vi "Func-엑셀 데이터를 그래프로 출력.vi"() -> ()   [LabVIEW 2015] (continued)
\n-40\t-40\t-28.416\n-40\t-40\t-28.418\n-40\t-40\t-28.417\n-40\t-40\t-28.42\n-40\t-40\t-28.421\n-40\t-40\t-28.421\n-40\t-40\t-28.429\n-40\t-40\t-28.43\n-40\t-40\t-28.434\n-40\t-40\t-28.438\n-40\t-40\t-28.439\n-40\t-40\t-28.439\n-40\t-40\t-28.438\n-40\t-40\t-28.443\n-40\t-40\t-28.445\n-40\t-40\t-28.446\n-40\t-40\t-28.45\n-40\t-40\t-28.455\n-40\t-40\t-28.458\n-40\t-40\t-28.458\n-40\t-40\t-28.46\n-40\t-40\t-28.465\n-40\t-40\t-28.466\n-40\t-40\t-28.466\n-40\t-40\t-28.471\n-40\t-40\t-28.47\n-40\t-40\t-28.475\n-40\t-40\t-28.474\n-40\t-40\t-28.476\n-40\t-40\t-28.478\n-40\t-40\t-28.48\n-40\t-40\t-28.48\n-40\t-40\t-28.479\n-40\t-40\t-28.485\n-40\t-40\t-28.484\n-40\t-40\t-28.488\n-40\t-40\t-28.494\n-40\t-40\t-28.498\n-40\t-40\t-28.499\n-40\t-40\t-28.499\n-40\t-40\t-28.502\n-40\t-40\t-28.504\n-40\t-40\t-28.504\n-40\t-40\t-28.507\n-40\t-40\t-28.508\n-40\t-40\t-28.514\n-40\t-40\t-28.518\n-40\t-40\t-28.52\n-40\t-40\t-28.523\n-40\t-40\t-28.524\n-40\t-40\t-28.53\n-40\t-40\t-28.534\n-40\t-40\t-28.536\n-40\t-40\t-28.539\n-40\t-40\t-28.543\n-40\t-40\t-28.544\n-40\t-40\t-28.544\n-40\t-40\t-28.542\n-40\t-40\t-28.542\n-40\t-40\t-28.542\n-40\t-40\t-28.544\n-40\t-40\t-28.548\n-40\t-40\t-28.55\n-40\t-40\t-28.553\n-40\t-40\t-28.552\n-40\t-40\t-28.554\n-40\t-40\t-28.555\n-40\t-40\t-28.557\n-40\t-40\t-28.557\n-40\t-40\t-28.559\n-40\t-40\t-28.564\n-40\t-40\t-28.57\n-40\t-40\t-28.57\n-40\t-40\t-28.57\n-40\t-40\t-28.574\n-40\t-40\t-28.578\n-40\t-40\t-28.58\n-40\t-40\t-28.577\n-40\t-40\t-28.581\n-40\t-40\t-28.585\n-40\t-40\t-28.586\n-40\t-40\t-28.588\n-40\t-40\t-28.587\n-40\t-40\t-28.593\n-40\t-40\t-28.593\n-40\t-40\t-28.593\n-40\t-40\t-28.594\n-40\t-40\t-28.596\n-40\t-40\t-28.602\n-40\t-40\t-28.605\n-40\t-40\t-28.611\n-40\t-40\t-28.614\n-40\t-40\t-28.617\n-40\t-40\t-28.621\n-40\t-40\t-28.62\n-40\t-40\t-28.62\n-40\t-40\t-28.618\n-40\t-40\t-28.618\n-40\t-40\t-28.62\n-40\t-40\t-28.62\n-40\t-40\t-28.625\n-40\t-40\t-28.629\n-40\t-40\t-28.634\n-40\t-40\t-28.635\n-40\t-40\t-28.636\n-40\t-40\t-28.639\n-40\t-40\t-28.639\n-40\t-40\t-28.643\n-40\t-40\t-28.643\n-40\t-40\t-28.646\n-40\t-40\t-28.65\n-40\t-40\t-28.652\n-40\t-40\t-28.653\n-40\t-40\t-28.654\n-40\t-40\t-28.656\n-40\t-40\t-28.655\n-40\t-40\t-28.655\n-40\t-40\t-28.657\n-40\t-40\t-28.658\n-40\t-40\t-28.662\n-40\t-40\t-28.662\n-40\t-40\t-28.666\n-40\t-40\t-28.67\n-40\t-40\t-28.674\n-40\t-40\t-28.676\n-40\t-40\t-28.677\n-40\t-40\t-28.679\n-40\t-40\t-28.684\n-40\t-40\t-28.687\n-40\t-40\t-28.687\n-40\t-40\t-28.688\n-40\t-40\t-28.692\n-40\t-40\t-28.691\n-40\t-40\t-28.69\n-40\t-40\t-28.692\n-40\t-40\t-28.695\n-40\t-40\t-28.697\n-40\t-40\t-28.695\n-40\t-40\t-28.7\n-40\t-40\t-28.703\n-40\t-40\t-28.708\n-40\t-40\t-28.708\n-40\t-40\t-28.709\n-40\t-40\t-28.716\n-40\t-40\t-28.72\n-40\t-40\t-28.72\n-40\t-40\t-28.718\n-40\t-40\t-28.721\n-40\t-40\t-28.724\n-40\t-40\t-28.726\n-40\t-40\t-28.728\n-40\t-40\t-28.731\n-40\t-40\t-28.733\n-40\t-40\t-28.732\n-40\t-40\t-28.731\n-40\t-40\t-28.731\n-40\t-40\t-28.73\n-40\t-40\t-28.732\n-40\t-40\t-28.736\n-40\t-40\t-28.739\n-40\t-40\t-28.742\n-40\t-40\t-28.745\n-40\t-40\t-28.746\n-40\t-40\t-28.748\n-40\t-40\t-28.75\n-40\t-40\t-28.751\n-40\t-40\t-28.752\n-40\t-40\t-28.754\n-40\t-40\t-28.755\n-40\t-40\t-28.757\n-40\t-40\t-28.758\n-40\t-40\t-28.761\n-40\t-40\t-28.762\n-40\t-40\t-28.764\n-40\t-40\t-28.767\n-40\t-40\t-28.769\n-40\t-40\t-28.772\n-40\t-40\t-28.774\n-40\t-40\t-28.778\n-40\t-40\t-28.775\n-40\t-40\t-28.778\n-40\t-40\t-28.78\n-40\t-40\t-28.781\n-40\t-40\t-28.781\n-40\t-40\t-28.784\n-40\t-40\t-28.791\n-40\t-40\t-28.793\n-40\t-40\t-28.793\n-40\t-40\t-28.799\n-40\t-40\t-28.8\n-40\t-40\t-28.801\n-40\t-40\t-28.802\n-40\t-40\t-28.804\n-40\t-40\t-28.803\n-40\t-40\t-28.805\n-40\t-40\t-28.806\n-40\t-40\t-28.807\n-40\t-40\t-28.808\n-40\t-40\t-28.809\n-40\t-40\t-28.813\n-40\t-40\t-28.812\n-40\t-40\t-28.815\n-40\t-40\t-28.819\n-40\t-40\t-28.823\n-40\t-40\t-28.821\n-40\t-40\t-28.824\n-40\t-40\t-28.826\n-40\t-40\t-28.827\n-40\t-40\t-28.829\n-40\t-40\t-28.831\n-40\t-40\t-28.837\n-40\t-40\t-28.839\n-40\t-40\t-28.844\n-40\t-40\t-28.845\n-40\t-40\t-28.848\n-40\t-40\t-28.85\n-40\t-40\t-28.848\n-40\t-40\t-28.848\n-40\t-40\t-28.846\n-40\t-40\t-28.85\n-40\t-40\t-28.851\n-40\t-40\t-28.848\n-40\t-40\t-28.851\n-40\t-40\t-28.851\n-40\t-40\t-28.855\n-40\t-40\t-28.855\n-40\t-40\t-28.856\n-40\t-40\t-28.861\n-40\t-40\t-28.862\n-40\t-40\t-28.867\n-40\t-40\t-28.868\n-40\t-40\t-28.871\n-40\t-40\t-28.871\n-40\t-40\t-28.873\n-40\t-40\t-28.873\n-40\t-40\t-28.874\n-40\t-40\t-28.876\n-40\t-40\t-28.875\n-40\t-40\t-28.879\n-40\t-40\t-28.881\n-40\t-40\t-28.881\n-40\t-40\t-28.886\n-40\t-40\t-28.888\n-40\t-40\t-28.892\n-40\t-40\t-28.891\n-40\t-40\t-28.893\n-40\t-40\t-28.899\n-40\t-40\t-28.895\n-40\t-40\t-28.897\n-40\t-40\t-28.899\n-40\t-40\t-28.905\n-40\t-40\t-28.906\n-40\t-40\t-28.905\n-40\t-40\t-28.911\n-40\t-40\t-28.911\n-40\t-40\t-28.911\n-40\t-40\t-28.911\n-40\t-40\t-28.913\n-40\t-40\t-28.918\n-40\t-40\t-28.918\n-40\t-40\t-28.919\n-40\t-40\t-28.919\n-40\t-40\t-28.923\n-40\t-40\t-28.924\n-40\t-40\t-28.924\n-40\t-40\t-28.926\n-40\t-40\t-28.929\n-40\t-40\t-28.932\n-40\t-40\t-28.931\n-40\t-40\t-28.931\n-40\t-40\t-28.932\n-40\t-40\t-28.935\n-40\t-40\t-28.936\n-40\t-40\t-28.938\n-40\t-40\t-28.941\n-40\t-40\t-28.943\n-40\t-40\t-28.945\n-40\t-40\t-28.943\n-40\t-40\t-28.945\n-40\t-40\t-28.943\n-40\t-40\t-28.942\n-40\t-40\t-28.943\n-40\t-40\t-28.943\n-40\t-40\t-28.948\n-40\t-40\t-28.946\n-40\t-40\t-28.948\n-40\t-40\t-28.955\n-40\t-40\t-28.955\n-40\t-40\t-28.958\n-40\t-40\t-28.959\n-40\t-40\t-28.965\n-40\t-40\t-28.969\n-40\t-40\t-28.966\n-40\t-40\t-28.971\n-40\t-40\t-28.971\n-40\t-40\t-28.974\n-40\t-40\t-28.974\n-40\t-40\t-28.974\n-40\t-40\t-28.971\n-40\t-40\t-28.968\n-40\t-40\t-28.971\n-40\t-40\t-28.974\n-40\t-40\t-28.975\n-40\t-40\t-28.977\n-40\t-40\t-28.987\n-40\t-40\t-28.994\n-40\t-40\t-28.995\n-40\t-40\t-28.996\n-40\t-40\t-28.997\n-40\t-40\t-29\n-40\t-40\t-29.003\n-40\t-40\t-29.003\n-40\t-40\t-29.003\n-40\t-40\t-29.002\n-40\t-40\t-29.004\n-40\t-40\t-29.003\n-40\t-40\t-29.003\n-40\t-40\t-29.005\n-40\t-40\t-29.006\n-40\t-40\t-29.01\n-40\t-40\t-29.009\n-40\t-40\t-29.01\n-40\t-40\t-29.009\n-40\t-40\t-29.007\n-40\t-40\t-29.007\n-40\t-40\t-29.011\n-40\t-40\t-29.015\n-40\t-40\t-29.018\n-40\t-40\t-29.02\n-40\t-40\t-29.022\n-40\t-40\t-29.024\n-40\t-40\t-29.024\n-40\t-40\t-29.024\n-40\t-40\t-29.025\n-40\t-40\t-29.03\n-40\t-40\t-29.035\n-40\t-40\t-29.036\n-40\t-40\t-29.033\n-40\t-40\t-29.031\n-40\t-40\t-29.031\n-40\t-40\t-29.034\n-40\t-40\t-29.032\n-40\t-40\t-29.033\n-40\t-40\t-29.037\n-40\t-40\t-29.04\n-40\t-40\t-29.043\n-40\t-40\t-29.047\n-40\t-40\t-29.047\n-40\t-40\t-29.048\n-40\t-40\t-29.053\n-40\t-40\t-29.055\n-40\t-40\t-29.055\n-40\t-40\t-29.055\n-40\t-40\t-29.059\n-40\t-40\t-29.062\n-40\t-40\t-29.063\n-40\t-40\t-29.066\n-40\t-40\t-29.067\n-40\t-40\t-29.067\n-40\t-40\t-29.066\n-40\t-40\t-29.066\n-40\t-40\t-29.071\n-40\t-40\t-29.075\n-40\t-40\t-29.075\n-40\t-40\t-29.076\n-40\t-40\t-29.079\n-40\t-40\t-29.082\n-40\t-40\t-29.079\n-40\t-40\t-29.078\n-40\t-40\t-29.079\n-40\t-40\t-29.079\n-40\t-40\t-29.08\n-40\t-40\t-29.08\n-40\t-40\t-29.08\n-40\t-40\t-29.081\n-40\t-40\t-29.084\n-40\t-40\t-29.09\n-40\t-40\t-29.091\n-40\t-40\t-29.091\n-40\t-40\t-29.098\n-40\t-40\t-29.096\n-40\t-40\t-29.099\n-40\t-40\t-29.096\n-40\t-40\t-29.098\n-40\t-40\t-29.1\n-40\t-40\t-29.101\n-40\t-40\t-29.106\n-40\t-40\t-29.108\n-40\t-40\t-29.111\n-40\t-40\t-29.114\n-40\t-40\t-29.117\n-40\t-40\t-29.12\n-40\t-40\t-29.119\n-40\t-40\t-29.121\n-40\t-40\t-29.123\n-40\t-40\t-29.121\n-40\t-40\t-29.12\n-40\t-40\t-29.121\n-40\t-40\t-29.123\n-40\t-40\t-29.12\n-40\t-40\t-29.123\n-40\t-40\t-29.126\n-40\t-40\t-29.128\n-40\t-40\t-29.129\n-40\t-40\t-29.129\n-40\t-40\t-29.132\n-40\t-40\t-29.133\n-40\t-40\t-29.134\n-40\t-40\t-29.136\n-40\t-40\t-29.138\n-40\t-40\t-29.137\n-40\t-40\t-29.139\n-40\t-40\t-29.142\n-40\t-40\t-29.141\n-40\t-40\t-29.142\n-40\t-40\t-29.143\n-40\t-40\t-29.146\n-40\t-40\t-29.145\n-40\t-40\t-29.146\n-40\t-40\t-29.148\n-40\t-40\t-29.148\n-40\t-40\t-29.151\n-40\t-40\t-29.15\n-40\t-40\t-29.152\n-40\t-40\t-29.149\n-40\t-40\t-29.153\n-40\t-40\t-29.157\n-40\t-40\t-29.155\n-40\t-40\t-29.161\n-40\t-40\t-29.163\n-40\t-40\t-29.165\n-40\t-40\t-29.165\n-40\t-40\t-29.164\n-40\t-40\t-29.166\n-40\t-40\t-29.162\n-40\t-40\t-29.161\n-40\t-40\t-29.166\n-40\t-40\t-29.168\n-40\t-40\t-29.169\n-40\t-40\t-29.171\n-40\t-40\t-29.175\n-40\t-40\t-29.177\n-40\t-40\t-29.177\n-40\t-40\t-29.18\n-40\t-40\t-29.182\n-40\t-40\t-29.184\n-40\t-40\t-29.186\n-40\t-40\t-29.187\n-40\t-40\t-29.186\n-40\t-40\t-29.186\n-40\t-40\t-29.19\n-40\t-40\t-29.193\n-40\t-40\t-29.191\n-40\t-40\t-29.191\n-40\t-40\t-29.197\n-40\t-40\t-29.197\n-40\t-40\t-29.196\n-40\t-40\t-29.196\n-40\t-40\t-29.2\n-40\t-40\t-29.2\n-40\t-40\t-29.2\n-40\t-40\t-29.199\n-40\t-40\t-29.199\n-40\t-40\t-29.202\n-40\t-40\t-29.202\n-40\t-40\t-29.206\n-40\t-40\t-29.205\n-40\t-40\t-29.208\n-40\t-40\t-29.208\n-40\t-40\t-29.209\n-40\t-40\t-29.211\n-40\t-40\t-29.211\n-40\t-40\t-29.213\n-40\t-40\t-29.215\n-40\t-40\t-29.22\n-40\t-40\t-29.221\n-40\t-40\t-29.226\n-40\t-40\t-29.226\n-40\t-40\t-29.23\n-40\t-40\t-29.231\n-40\t-40\t-29.229\n-40\t-40\t-29.229\n-40\t-40\t-29.226\n-40\t-40\t-29.229\n-40\t-40\t-29.23\n-40\t-40\t-29.232\n-40\t-40\t-29.233\n-40\t-40\t-29.238\n-40\t-40\t-29.24\n-40\t-40\t-29.24\n-40\t-40\t-29.241\n-40\t-40\t-29.241\n-40\t-40\t-29.241\n-40\t-40\t-29.243\n-40\t-40\t-29.243\n-40\t-40\t-29.247\n-40\t-40\t-29.251\n-40\t-40\t-29.251\n-40\t-40\t-29.254\n-40\t-40\t-29.252\n-40\t-40\t-29.252\n-40\t-40\t-29.253\n-40\t-40\t-29.252\n-40\t-40\t-29.254\n-40\t-40\t-29.254\n-40\t-40\t-29.259\n-40\t-40\t-29.262\n-40\t-40\t-29.26\n-40\t-40\t-29.259\n-40\t-40\t-29.259\n-40\t-40\t-29.261\n-40\t-40\t-29.26\n-40\t-40\t-29.261\n-40\t-40\t-29.262\n-40\t-40\t-29.267\n-40\t-40\t-29.27\n-40\t-40\t-29.27\n-40\t-40\t-29.27\n-40\t-40\t-29.273\n-40\t-40\t-29.273\n-40\t-40\t-29.273\n-40\t-40\t-29.275\n-40\t-40\t-29.277\n-40\t-40\t-29.279\n-40\t-40\t-29.277\n-40\t-40\t-29.284\n-40\t-40\t-29.286\n-40\t-40\t-29.285\n-40\t-40\t-29.288\n-40\t-40\t-29.291\n-40\t-40\t-29.289\n-40\t-40\t-29.288\n-40\t-40\t-29.284\n-40\t-40\t-29.284\n-40\t-40\t-29.283\n-40\t-40\t-29.282\n-40\t-40\t-29.284\n-40\t-40\t-29.286\n-40\t-40\t-29.29\n-40\t-40\t-29.294\n-40\t-40\t-29.298\n-40\t-40\t-29.302\n-40\t-40\t-29.303\n-40\t-40\t-29.302\n-40\t-40\t-29.301\n-40\t-40\t-29.3\n-40\t-40\t-29.297\n-40\t-40\t-29.295\n-40\t-40\t-29.297\n-40\t-40\t-29.3\n-40\t-40\t-29.307\n-40\t-40\t-29.307\n-40\t-40\t-29.309\n-40\t-40\t-29.312\n-40\t-40\t-29.313\n-40\t-40\t-29.312\n-40\t-40\t-29.309\n-40\t-40\t-29.313\n-40\t-40\t-29.314\n-40\t-40\t-29.318\n-40\t-40\t-29.32\n-40\t-40\t-29.32\n-40\t-40\t-29.325\n-40\t-40\t-29.325\n-40\t-40\t-29.327\n-40\t-40\t-29.327\n-40\t-40\t-29.329\n-40\t-40\t-29.33\n-40\t-40\t-29.327\n-40\t-40\t-29.326\n-40\t-40\t-29.325\n-40\t-40\t-29.326\n-40\t-40\t-29.328\n-40\t-40\t-29.329\n-40\t-40\t-29.332\n-40\t-40\t-29.332\n-40\t-40\t-29.337\n-40\t-40\t-29.339\n-40\t-40\t-29.339\n-40\t-40\t-29.34\n-40\t-40\t-29.343\n-40\t-40\t-29.347\n-40\t-40\t-29.345\n-40\t-40\t-29.346\n-40\t-40\t-29.348\n-40\t-40\t-29.351\n-40\t-40\t-29.349\n-40\t-40\t-29.346\n-40\t-40\t-29.347\n-40\t-40\t-29.349\n-40\t-40\t-29.349\n-40\t-40\t-29.35\n-40\t-40\t-29.356\n-40\t-40\t-29.359\n-40\t-40\t-29.357\n-40\t-40\t-29.356\n-40\t-40\t-29.355\n-40\t-40\t-29.358\n-40\t-40\t-29.359\n-40\t-40\t-29.362\n-40\t-40\t-29.365\n-40\t-40\t-29.37\n-40\t-40\t-29.368\n-40\t-40\t-29.365\n-40\t-40\t-29.364\n-40\t-40\t-29.365\n-40\t-40\t-29.369\n-40\t-40\t-29.363\n-40\t-40\t-29.366\n-40\t-40\t-29.367\n-40\t-40\t-29.37\n-40\t-40\t-29.37\n-40\t-40\t-29.37\n-40\t-40\t-29.376\n-40\t-40\t-29.378\n-40\t-40\t-29.38\n-40\t-40\t-29.383\n-40\t-40\t-29.385\n-40\t-40\t-29.381\n-40\t-40\t-29.382\n-40\t-40\t-29.385\n-40\t-40\t-29.385\n-40\t-40\t-29.384\n-40\t-40\t-29.383\n-40\t-40\t-29.386\n-40\t-40\t-29.386\n-40\t-40\t-29.386\n-40\t-40\t-29.387\n-40\t-40\t-29.389\n-40\t-40\t-29.39\n-40\t-40\t-29.392\n-40\t-40\t-29.393\n-40\t-40\t-29.393\n-40\t-40\t-29.396\n-40\t-40\t-29.4\n-40\t-40\t-29.404\n-40\t-40\t-29.401\n-40\t-40\t-29.401\n-40\t-40\t-29.404\n-40\t-40\t-29.401\n-40\t-40\t-29.398\n-40\t-40\t-29.397\n-40\t-40\t-29.399\n-40\t-40\t-29.402\n-40\t-40\t-29.4\n-40\t-40\t-29.405\n-40\t-40\t-29.41\n-40\t-40\t-29.413\n-40\t-40\t-29.413\n-40\t-40\t-29.413\n-40\t-40\t-29.413\n-40\t-40\t-29.411\n-40\t-40\t-29.41\n-40\t-40\t-29.409\n-40\t-40\t-29.41\n-40\t-40\t-29.414\n-40\t-40\t-29.415\n-40\t-40\t-29.416\n-40\t-40\t-29.418\n-40\t-40\t-29.419\n-40\t-40\t-29.421\n-40\t-40\t-29.42\n-40\t-40\t-29.423\n-40\t-40\t-29.424\n-40\t-40\t-29.422\n-40\t-40\t-29.423\n-40\t-40\t-29.424\n-40\t-40\t-29.423\n-40\t-40\t-29.423\n-40\t-40\t-29.424\n-40\t-40\t-29.43\n-40\t-40\t-29.431\n-40\t-40\t-29.43\n-40\t-40\t-29.434\n-40\t-40\t-29.435\n-40\t-40\t-29.438\n-40\t-40\t-29.436\n-40\t-40\t-29.44\n-40\t-40\t-29.441\n-40\t-40\t-29.441\n-40\t-40\t-29.444\n-40\t-40\t-29.442\n-40\t-40\t-29.442\n-40\t-40\t-29.441\n-40\t-40\t-29.443\n-40\t-40\t-29.446\n-40\t-40\t-29.446\n-40\t-40\t-29.447\n-40\t-40\t-29.454\n-40\t-40\t-29.452\n-40\t-40\t-29.452\n-40\t-40\t-29.454\n-40\t-40\t-29.454\n-40\t-40\t-29.456\n-40\t-40\t-29.452\n-40\t-40\t-29.452\n-40\t-40\t-29.455\n-40\t-40\t-29.455\n-40\t-40\t-29.453\n-40\t-40\t-29.453\n-40\t-40\t-29.457\n-40\t-40\t-29.46\n-40\t-40\t-29.459\n-40\t-40\t-29.462\n-40\t-40\t-29.464\n-40\t-40\t-29.464\n-40\t-40\t-29.466\n-40\t-40\t-29.467\n-40\t-40\t-29.468\n-40\t-40\t-29.47\n-40\t-40\t-29.471\n-40\t-40\t-29.474\n-40\t-40\t-29.474\n-40\t-40\t-29.473\n-40\t-40\t-29.476\n-40\t-40\t-29.472\n-40\t-40\t-29.473\n-40\t-40\t-29.472\n-40\t-40\t-29.471\n-40\t-40\t-29.473\n-40\t-40\t-29.473\n-40\t-40\t-29.475\n-40\t-40\t-29.477\n-40\t-40\t-29.477\n-40\t-40\t-29.475\n-40\t-40\t-29.476\n-40\t-40\t-29.475\n-40\t-40\t-29.474\n-40\t-40\t-29.474\n-40\t-40\t-29.476\n-40\t-40\t-29.481\n-40\t-40\t-29.484\n-40\t-40\t-29.485\n-40\t-40\t-29.49\n-40\t-40\t-29.493\n-40\t-40\t-29.492\n-40\t-40\t-29.496\n-40\t-40\t-29.498\n-40\t-40\t-29.498\n-40\t-40\t-29.5\n-40\t-40\t-29.5\n-40\t-40\t-29.501\n-40\t-40\t-29.496\n-40\t-40\t-29.493\n-40\t-40\t-29.495\n-40\t-40\t-29.495\n-40\t-40\t-29.494\n-40\t-40\t-29.496\n-40\t-40\t-29.498\n-40\t-40\t-29.499\n-40\t-40\t-29.498\n-40\t-40\t-29.499\n-40\t-40\t-29.5\n-40\t-40\t-29.502\n-40\t-40\t-29.501\n-40\t-40\t-29.502\n-40\t-40\t-29.501\n-40\t-40\t-29.5\n-40\t-40\t-29.5\n-40\t-40\t-29.501\n-40\t-40\t-29.502\n-40\t-40\t-29.507\n-40\t-40\t-29.51\n-40\t-40\t-29.509\n-40\t-40\t-29.511\n-40\t-40\t-29.512\n-40\t-40\t-29.513\n-40\t-40\t-29.51\n-40\t-40\t-29.511\n-40\t-40\t-29.512\n-40\t-40\t-29.514\n-40\t-40\t-29.514\n-40\t-40\t-29.516\n-40\t-40\t-29.516\n-40\t-40\t-29.516\n-40\t-40\t-29.523\n-40\t-40\t-29.521\n-40\t-40\t-29.521\n-40\t-40\t-29.523\n-40\t-40\t-29.524\n-40\t-40\t-29.526\n-40\t-40\t-29.522\n-40\t-40\t-29.522\n-40\t-40\t-29.526\n-40\t-40\t-29.529\n-40\t-40\t-29.531\n-40\t-40\t-29.534\n-40\t-40\t-29.536\n-40\t-40\t-29.54\n-40\t-40\t-29.539\n-40\t-40\t-29.539\n-40\t-40\t-29.543\n-40\t-40\t-29.536\n-40\t-40\t-29.539\n-40\t-40\t-29.542\n-40\t-40\t-29.542\n-40\t-40\t-29.542\n-40\t-40\t-29.541\n-40\t-40\t-29.543\n-40\t-40\t-29.539\n-40\t-40\t-29.538\n-40\t-40\t-29.541\n-40\t-40\t-29.54\n-40\t-40\t-29.54\n-40\t-40\t-29.544\n-40\t-40\t-29.549\n-40\t-40\t-29.55\n-40\t-40\t-29.548\n-40\t-40\t-29.552\n-40\t-40\t-29.551\n-40\t-40\t-29.553\n-40\t-40\t-29.55\n-40\t-40\t-29.552\n-40\t-40\t-29.554\n-40\t-40\t-29.554\n-40\t-40\t-29.555\n-40\t-40\t-29.554\n-40\t-40\t-29.558\n-40\t-40\t-29.561\n-40\t-40\t-29.56\n-40\t-40\t-29.562\n-40\t-40\t-29.561\n-40\t-40\t-29.56\n-40\t-40\t-29.556\n-40\t-40\t-29.556\n-40\t-40\t-29.556\n-40\t-40\t-29.556\n-40\t-40\t-29.558\n-40\t-40\t-29.559\n-40\t-40\t-29.561\n-40\t-40\t-29.557\n-40\t-40\t-29.56\n-40\t-40\t-29.558\n-40\t-40\t-29.561\n-40\t-40\t-29.563\n-40\t-40\t-29.566\n-40\t-40\t-29.57\n-40\t-40\t-29.57\n-40\t-40\t-29.573\n-40\t-40\t-29.575\n-40\t-40\t-29.576\n-40\t-40\t-29.573\n-40\t-40\t-29.573\n-40\t-40\t-29.571\n-40\t-40\t-29.567\n-40\t-40\t-29.568\n-40\t-40\t-29.568\n-40\t-40\t-29.572\n-40\t-40\t-29.578\n-40\t-40\t-29.58\n-40\t-40\t-29.587\n-40\t-40\t-29.585\n-40\t-40\t-29.587\n-40\t-40\t-29.586\n-40\t-40\t-29.584\n-40\t-40\t-29.585\n-40\t-40\t-29.584\n-40\t-40\t-29.586\n-40\t-40\t-29.585\n-40\t-40\t-29.584\n-40\t-40\t-29.582\n-40\t-40\t-29.581\n-40\t-40\t-29.582\n-40\t-40\t-29.585\n-40\t-40\t-29.586\n-40\t-40\t-29.591\n-40\t-40\t-29.598\n-40\t-40\t-29.597\n-40\t-40\t-29.598\n-40\t-40\t-29.599\n-40\t-40\t-29.601\n-40\t-40\t-29.6\n-40\t-40\t-29.598\n-40\t-40\t-29.601\n-40\t-40\t-29.602\n-40\t-40\t-29.602\n-40\t-40\t-29.601\n-40\t-40\t-29.601\n-40\t-40\t-29.602\n-40\t-40\t-29.603\n-40\t-40\t-29.603\n-40\t-40\t-29.605\n-40\t-40\t-29.607\n-40\t-40\t-29.606\n-40\t-40\t-29.604\n-40\t-40\t-29.607\n-40\t-40\t-29.606\n-40\t-40\t-29.603\n-40\t-40\t-29.602\n-40\t-40\t-29.604\n-40\t-40\t-29.612\n-40\t-40\t-29.611\n-40\t-40\t-29.613\n-40\t-40\t-29.616\n-40\t-40\t-29.617\n-40\t-40\t-29.618\n-40\t-40\t-29.616\n-40\t-40\t-29.615\n-40\t-40\t-29.613\n-40\t-40\t-29.616\n-40\t-40\t-29.616\n-40\t-40\t-29.617\n-40\t-40\t-29.618\n-40\t-40\t-29.618\n-40\t-40\t-29.62\n-40\t-40\t-29.62\n-40\t-40\t-29.623\n-40\t-40\t-29.622\n-40\t-40\t-29.621\n-40\t-40\t-29.625\n-40\t-40\t-29.624\n-40\t-40\t-29.621\n-40\t-40\t-29.618\n-40\t-40\t-29.62\n-40\t-40\t-29.623\n-40\t-40\t-29.621\n-40\t-40\t-29.624\n-40\t-40\t-29.629\n-40\t-40\t-29.633\n-40\t-40\t-29.634\n-40\t-40\t-29.631\n-40\t-40\t-29.633\n-40\t-40\t-29.633\n-40\t-40\t-29.631\n-40\t-40\t-29.632\n-40\t-40\t-29.634\n-40\t-40\t-29.635\n-40\t-40\t-29.635\n-40\t-40\t-29.634\n-40\t-40\t-29.636\n-40\t-40\t-29.632\n-40\t-40\t-29.63\n-40\t-40\t-29.629\n-40\t-40\t-29.632\n-40\t-40\t-29.635\n-40\t-40\t-29.634\n-40\t-40\t-29.636\n-40\t-40\t-29.639\n-40\t-40\t-29.64\n-40\t-40\t-29.637\n-40\t-40\t-29.637\n-40\t-40\t-29.641\n-40\t-40\t-29.643\n-40\t-40\t-29.639\n-40\t-40\t-29.641\n-40\t-40\t-29.644\n-40\t-40\t-29.647\n-40\t-40\t-29.649\n-40\t-40\t-29.65\n-40\t-40\t-29.653\n-40\t-40\t-29.655\n-40\t-40\t-29.657\n-40\t-40\t-29.652\n-40\t-40\t-29.649\n-40\t-40\t-29.65\n-40\t-40\t-29.65\n-40\t-40\t-29.654\n-40\t-40\t-29.65\n-40\t-40\t-29.654\n-40\t-40\t-29.659\n-40\t-40\t-29.659\n-40\t-40\t-29.659\n-40\t-40\t-29.655\n-40\t-40\t-29.657\n-40\t-40\t-29.658\n-40\t-40\t-29.658\n-40\t-40\t-29.656\n-40\t-40\t-29.658\n-40\t-40\t-29.659\n-40\t-40\t-29.659\n-40\t-40\t-29.66\n-40\t-40\t-29.658\n-40\t-40\t-29.661\n-40\t-40\t-29.662\n-40\t-40\t-29.667\n-40\t-40\t-29.666\n-40\t-40\t-29.668\n-40\t-40\t-29.671\n-40\t-40\t-29.67\n-40\t-40\t-29.67\n-40\t-40\t-29.668\n-40\t-40\t-29.669\n-40\t-40\t-29.667\n-40\t-40\t-29.667\n-40\t-40\t-29.669\n-40\t-40\t-29.672\n-40\t-40\t-29.673\n-40\t-40\t-29.676\n-40\t-40\t-29.677\n-40\t-40\t-29.678\n-40\t-40\t-29.677\n-40\t-40\t-29.676\n-40\t-40\t-29.678\n-40\t-40\t-29.678\n-40\t-40\t-29.679\n-40\t-40\t-29.683\n-40\t-40\t-29.682\n-40\t-40\t-29.682\n-40\t-40\t-29.68\n-40\t-40\t-29.683\n-40\t-40\t-29.681\n-40\t-40\t-29.679\n-40\t-40\t-29.678\n-40\t-40\t-29.678\n-40\t-40\t-29.683\n-40\t-40\t-29.683\n-40\t-40\t-29.686\n-40\t-40\t-29.689\n-40\t-40\t-29.69\n-40\t-40\t-29.69\n-40\t-40\t-29.689\n-40\t-40\t-29.689\n-40\t-40\t-29.689\n-40\t-40\t-29.686\n-40\t-40\t-29.689\n-40\t-40\t-29.69\n-40\t-40\t-29.689\n-40\t-40\t-29.691\n-40\t-40\t-29.691\n-40\t-40\t-29.692\n-40\t-40\t-29.689\n-40\t-40\t-29.694\n-40\t-40\t-29.693\n-40\t-40\t-29.691\n-40\t-40\t-29.689\n-40\t-40\t-29.691\n-40\t-40\t-29.692\n-40\t-40\t-29.692\n-40\t-40\t-29.695\n-40\t-40\t-29.697\n-40\t-40\t-29.7\n-40\t-40\t-29.703\n-40\t-40\t-29.702\n25\t-40\t-30.028\n25\t-40.02\t-30.027\n25\t-40.01\t-30.025\n25\t-40.01\t-30.029\n25\t-40.01\t-30.029\n25\t-40\t-30.036\n25\t-39.98\t-30.034\n25\t-39.97\t-30.033\n25\t-39.95\t-30.03\n25\t-39.93\t-30.031\n25\t-39.89\t-30.032\n25\t-39.85\t-30.032\n25\t-39.79\t-30.032\n25\t-39.73\t-30.03\n25\t-39.65\t-30.035\n25\t-39.58\t-30.036\n25\t-39.49\t-30.039\n25\t-39.4\t-30.04\n25\t-39.29\t-30.037\n25\t-39.19\t-30.038\n25\t-39.07\t-30.033\n25\t-38.95\t-30.039\n25\t-38.82\t-30.038\n25\t-38.68\t-30.04\n25\t-38.55\t-30.038\n
